vi "_Get Sheets.vi"(8 "error in":errorcluster, 11 "SpreadsheetDocument in":refnum<k24>) -> (0 "error out":errorcluster, 2 "Sheets":refnum<k24>, 3 "SpreadsheetDocument out":refnum<k24>)   [LabVIEW 2021, in "Open Xml.lvlib"]
uses:
  Open Xml.lvlib
  D:/git/Open-Xml-LabVIEW/dll/DocumentFormat.OpenXml.dll
  dll/DocumentFormat.OpenXml.dll
  D:/git/Open-Xml-LabVIEW/dll/DocumentFormat.OpenXml.Framework.dll
  dll/DocumentFormat.OpenXml.Framework.dll
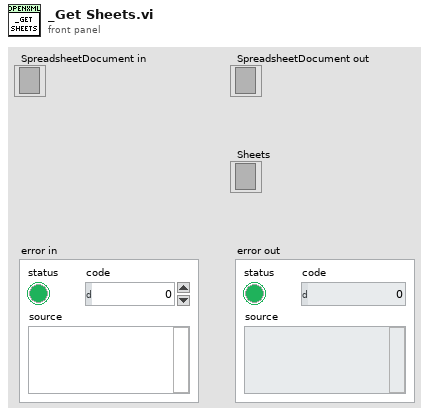
[diagram p1: front panel]
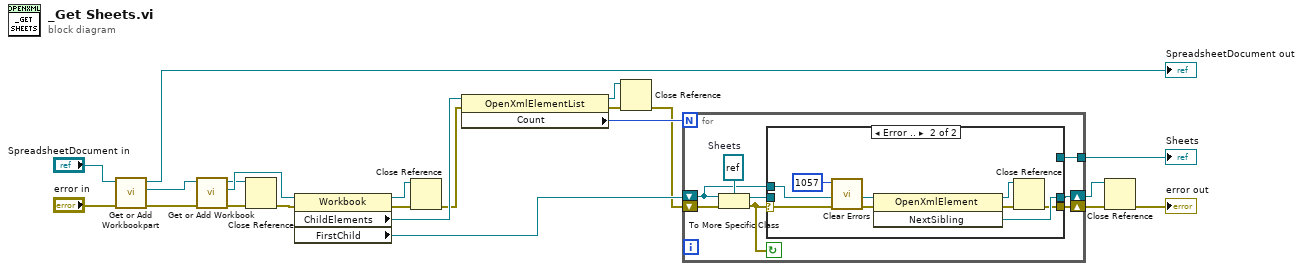
[diagram p0: block diagram]
diagram:
  n1 = call "Get or Add Workbookpart.vi"("error in"="error in", "SpreadsheetDocument"="SpreadsheetDocument in") -> ("error out"=w6:errorcluster, "WorkbookPart"=w4:refnum<k24>, "SpreadsheetDocument out"=→"SpreadsheetDocument out":refnum<k24>)  [unwired: 7 in]
  n2 = call "Get or Add Workbook.vi"("error in"=w6, "Workbookpart in"=w4) -> ("error out"=w12:errorcluster, "Workbook"=w3:refnum<k24>, "Workbookpart out"=w1:refnum<k24>)  [unwired: 7 in]
  n3 = Close Reference(reference=w1, error in (no error)=w12) -> (error out=w2:errorcluster)
  n4 = property class="Workbook"(reference=w3, error in=w2) -> (reference out=w10:refnum<k24>, error out=w17:errorcluster, "ChildElements"=w21:refnum<k24>, "FirstChild"=w22:refnum<k24>)
  n5 = Close Reference(reference=w10, error in (no error)=w17) -> (error out=w11:errorcluster)
  n6 = property class="OpenXmlElementList"(reference=w21, error in=w11) -> (reference out=w8:refnum<k24>, error out=w16:errorcluster, "Count"=w20:i32)
  n7 = Close Reference(reference=w8, error in (no error)=w16) -> (error out=w9:errorcluster)
  n8 = for {
    N: w20 -> [_]
    shift-right: [w28] -> w14
    shift-left: w22 -> [w26]
    tunnel: [w24] -> w13
    shift-right: [w27] -> w18
    shift-left: w9 -> [w29]
    stop <- w25 continue-if-true
    w30 = refnum<k24> refnum  # Sheets
    n9 = To More Specific Class(target class=w30, reference=w26, error in=w29) -> (specific class reference=w23:refnum<k24>, error out=w25:errorcluster)
    n10 = case shown="Error .." w25 {
      selector: w25 -> [w32 w40]
      tunnel: w23 -> [w31 _]
      tunnel: [_ w39] -> w28
      tunnel: [w32 w33] -> w27
      tunnel: w26 -> [_ w38]
      tunnel: [w31 _] -> w24
      frame No Error {
      }
      frame Error {
        n11 = call <vilib>:"Clear Errors.vi"("error in (no error)"=w40, "specific error code to clear (0: all)"=1057) -> ("error out"=w37:errorcluster)  [unwired: 4 in, 1 out]
        n12 = invoke class="OpenXmlElement" method="NextSibling"(reference=w38, error in=w37) -> (reference out=w35:refnum<k24>, error out=w34:errorcluster, "NextSibling"=w39:refnum<k24>)  [unwired: 1 in]
        n13 = Close Reference(reference=w35, error in (no error)=w34) -> (error out=w33:errorcluster)
      }
    }
  }
  "Sheets" <- w13
  n14 = Close Reference(reference=w14, error in (no error)=w18) -> (error out=→"error out":errorcluster)
